vi "Average_temp_sensor.vi"() -> ()   [LabVIEW 2019]
uses:
  <vilib>/numeric/Random Number (Range) DBL.vi
panel:
  in  "stop":bool
  out "Average Body \nTemperature":dbl
  out "Thermometer":dbl(slide) scale=34.0..40.0
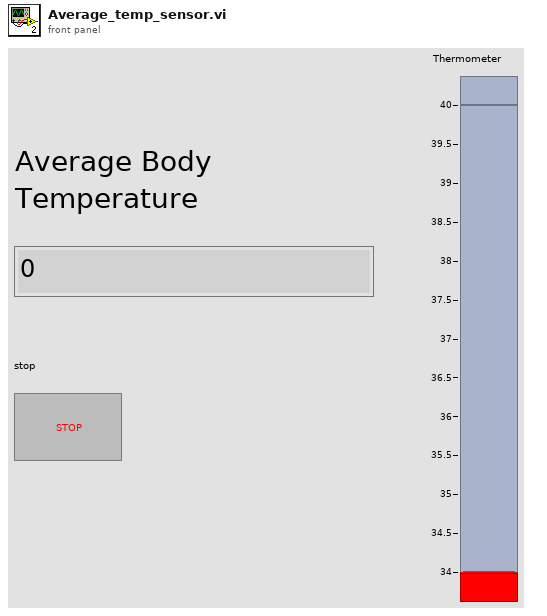
[diagram p1: front panel]
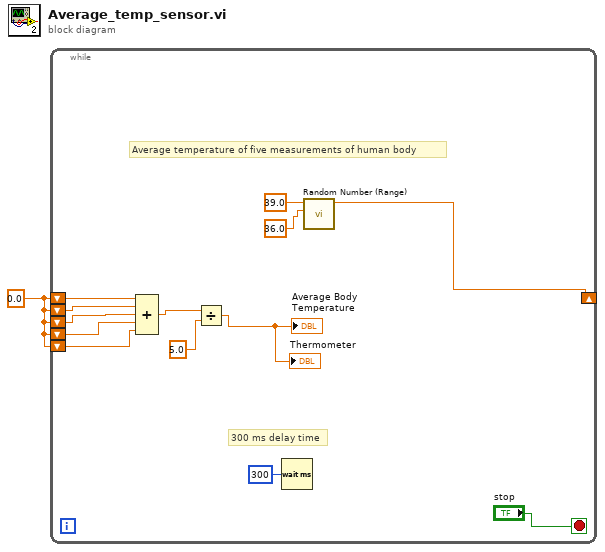
[diagram p0: block diagram]
diagram:
  w1 = 0.0
  n1 = while {
    shift-right: [w4] -> _
    shift-left: w1 -> [w14]
    shift-left: w1 -> [w13]
    shift-left: w1 -> [w12]
    shift-left: w1 -> [w11]
    shift-left: w1 -> [w10]
    stop <- "stop" stop-if-true
    # "300 ms delay time"
    # "Average temperature of five measurements of human body"
    n2 = Compound Arithmetic op=ADD(w14, w13, w12, w11, w10) -> (w9:dbl)
    n3 = Divide(x=w9, y=5.0) -> (x/y=→"Thermometer" →"Average Body \nTemperature":dbl)
    n4 = Wait (ms)(milliseconds to wait=u32 300) -> ()  [unwired: 1 out]
    n5 = call-poly <vilib>:"Random Number (Range).vi"("lower bound (0)"=36.0 ("upper bound (100)"), "upper bound (100)"=39.0) -> ("number"=w4:dbl)  [unwired: 9 in]
  }
